vi "Set AO.vi"(0 "Module Ref":refnum<class "Modbus Master.lvclass">, 5 "Analogue Voltage Out":dbl, 7 "Voltage Output range":T1 items=["+-5V"=142, "+-10V"=143, "0~5V"=147, "0~10V"=148], 9 "Channel":enum16{"AO0.V+", "AO1.V+", "AO2.V+", "AO3.V+"}(ring), 11 "error in (no error)":errorcluster) -> (4 "Modbus master out":refnum<class "Modbus Master.lvclass">, 15 "error out":errorcluster)   [LabVIEW 2024]
doc: "Set digital output states."
uses:
  <vilib>/NI/Modbus Library/API/Master/Modbus Master.lvclass
  Support VIs/AO Voltage Range.ctl
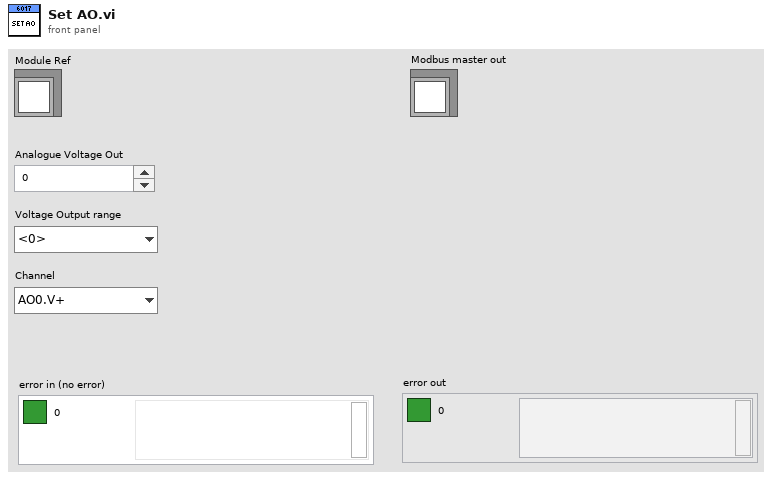
[diagram p1: front panel]
types:
  T1 = typedef "AO Voltage Range.ctl" = u16
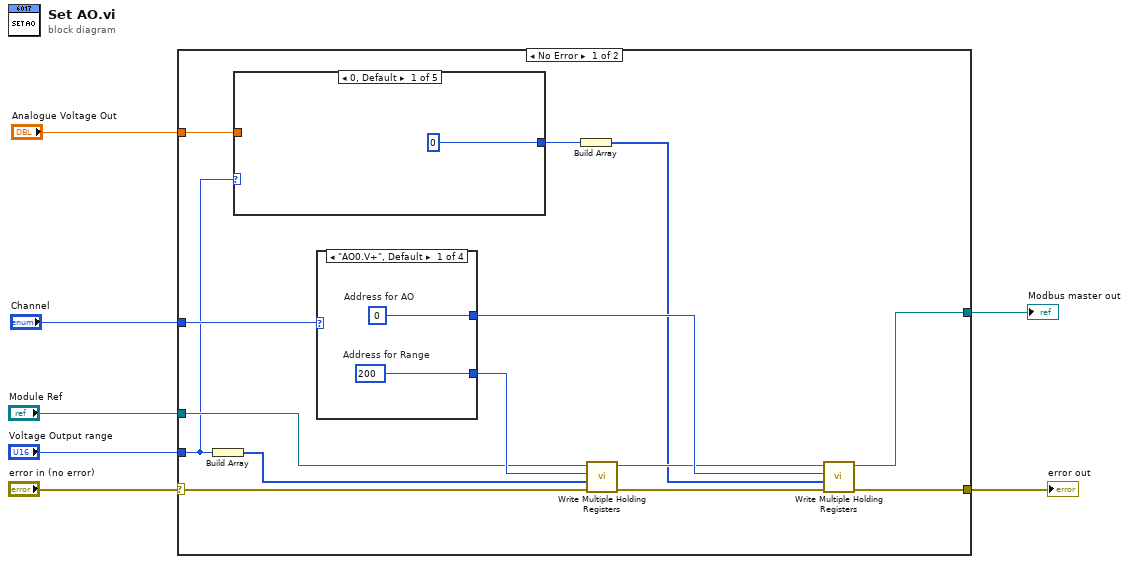
[diagram p0: block diagram]
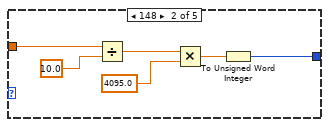
[diagram p2: hidden frame]
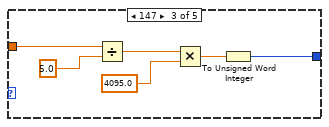
[diagram p3: hidden frame]
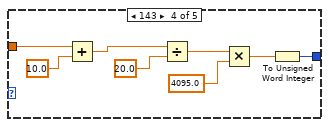
[diagram p4: hidden frame]
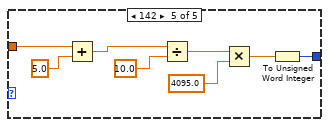
[diagram p5: hidden frame]
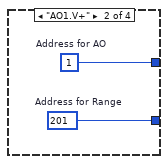
[diagram p6: hidden frame]
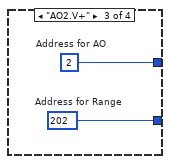
[diagram p7: hidden frame]
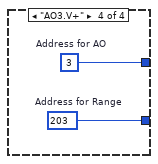
[diagram p8: hidden frame]
diagram:
  n1 = case shown="No Error" "error in (no error)" {
    selector: "error in (no error)" -> [w19 w59]
    tunnel: "Module Ref" -> [w14 w60]
    tunnel: [w21 w59] -> w5
    tunnel: [w20 w60] -> w4
    tunnel: "Channel" -> [w17 _]
    tunnel: "Voltage Output range" -> [w10 _]
    tunnel: "Analogue Voltage Out" -> [w11 _]
    frame No Error {
      n2 = Build Array(w10) -> (w12:T1[])
      n3 = case shown="0, Default" w10 {
        tunnel: w11 -> [_ w28 w34 w37 w45]
        tunnel: [u16 0 w23 w29 w38 w46] -> w9
        frame 0, Default {
        }
        frame 148 {
          n4 = Divide(x=w28, y=10.0) -> (x/y=w26:dbl)
          n5 = Multiply(x=w26, y=4095.0) -> (x*y=w24:dbl)
          n6 = To Unsigned Word Integer(number=w24) -> (unsigned 16bit integer=w23:u16)
        }
        frame 147 {
          n7 = Divide(x=w34, y=5.0) -> (x/y=w32:dbl)
          n8 = Multiply(x=w32, y=4095.0) -> (x*y=w30:dbl)
          n9 = To Unsigned Word Integer(number=w30) -> (unsigned 16bit integer=w29:u16)
        }
        frame 143 {
          n10 = Add(x=w37, y=10.0) -> (x+y=w35:dbl)
          n11 = Divide(x=w35, y=20.0) -> (x/y=w41:dbl)
          n12 = Multiply(x=w41, y=4095.0) -> (x*y=w39:dbl)
          n13 = To Unsigned Word Integer(number=w39) -> (unsigned 16bit integer=w38:u16)
        }
        frame 142 {
          n14 = Add(x=w45, y=5.0) -> (x+y=w43:dbl)
          n15 = Divide(x=w43, y=10.0) -> (x/y=w49:dbl)
          n16 = Multiply(x=w49, y=4095.0) -> (x*y=w47:dbl)
          n17 = To Unsigned Word Integer(number=w47) -> (unsigned 16bit integer=w46:u16)
        }
      }
      n18 = case shown="\"AO0.V+\", Default" w17 {
        tunnel: [w52 w53 w56 w58] -> w16
        tunnel: [w51 w54 w55 w57] -> w15
        frame "AO0.V+", Default {
          w51 = u16 200  # Address for Range
          w52 = u16 0  # Address for AO
        }
        frame "AO1.V+" {
          w54 = u16 201  # Address for Range
          w53 = u16 1  # Address for AO
        }
        frame "AO2.V+" {
          w55 = u16 202  # Address for Range
          w56 = u16 2  # Address for AO
        }
        frame "AO3.V+" {
          w57 = u16 203  # Address for Range
          w58 = u16 3  # Address for AO
        }
      }
      n19 = Build Array(w9) -> (w8:u16[])
      n20 = call-dynamic "Write Multiple Holding Registers.vi"("error in"=w19, "registers to write"=w12, "starting address"=w15, "Modbus master in"=w14) -> ("error out"=w18:errorcluster, "Modbus master out"=w13:refnum<class "Modbus Master.lvclass">)  [unwired: 6 in]
      n21 = call-dynamic "Write Multiple Holding Registers.vi"("error in"=w18, "registers to write"=w8, "starting address"=w16, "Modbus master in"=w13) -> ("error out"=w21:errorcluster, "Modbus master out"=w20:refnum<class "Modbus Master.lvclass">)  [unwired: 6 in]
    }
    frame Error {
    }
  }
  "error out" <- w5
  "Modbus master out" <- w4
